vi "Set Class Log_File.vi"(8 "error in (no error)":errorcluster caption="entrée d'erreur (pas d'erreur)", 10 "Library Log_File.lvlib:Class Log_File Altyor.lvclass":refnum<class "Class Log_File Altyor.lvclass">, 11 "Class Instrument Log_File en entrée":refnum<class "Class Instrument Log_File.lvclass">) -> (0 "error out":errorcluster caption="sortie d'erreur", 3 "Class Instrument Log_File en sortie":refnum<class "Class Instrument Log_File.lvclass">)   [LabVIEW 2020, in "Library Instrument & Equipement.lvlib" / "Library Instruments.lvlib" / "Class Instrument Log_File.lvclass"]
uses:
  Class Instrument Log_File.lvclass
  Log File/Class Log_File Altyor/Class Log_File Altyor.lvclass
  Class Instrument Log_File.lvclass/Class Instrument Log_File.ctl
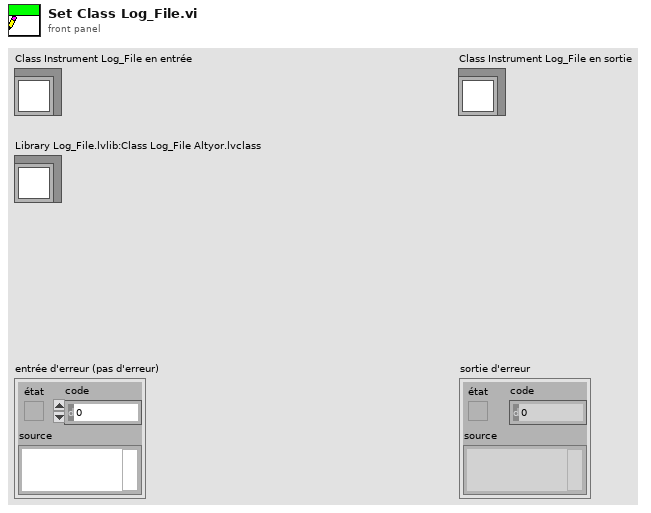
[diagram p1: front panel]
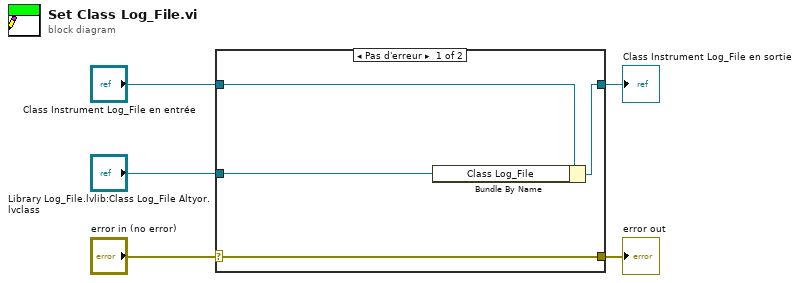
[diagram p0: block diagram]
diagram:
  n1 = case shown="Pas d'erreur" "error in (no error)" {
    selector: "error in (no error)" -> [w9 w10]
    tunnel: [w9 w10] -> w4
    tunnel: [w7 w11] -> w2
    tunnel: "Class Instrument Log_File en entrée" -> [w8 w11]
    tunnel: "Library Log_File.lvlib:Class Log_File Altyor.lvclass" -> [w6 _]
    frame No Error {
      n2 = Bundle By Name(cluster=w8, "Class Log_File"=w6) -> (w7:refnum<class "Class Instrument Log_File.lvclass">)
    }
    frame Error {
    }
  }
  "error out" <- w4
  "Class Instrument Log_File en sortie" <- w2
